vi "Subtract (Elementwise) - R,RM.vi"(1 "Real Matrix A":T1, 2 "Real Scalar c":dbl) -> (0 "c - A":T1)   [LabVIEW 2018, in "NI_Matrix.lvlib"]
doc: "Computes the difference of the inputs."
uses:
  NI_Matrix.lvlib
  RealMatrix.ctl
  Matrix To Array - RM.vi
  Array To Matrix - RA2.vi
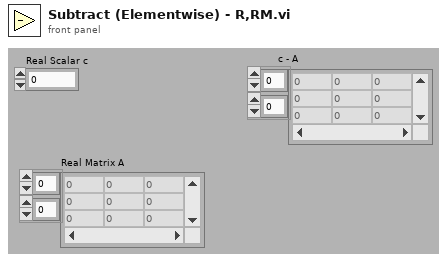
[diagram p1: front panel]
types:
  T1 = typedef "NI_Matrix.lvlib/RealMatrix.ctl" = dbl[][]
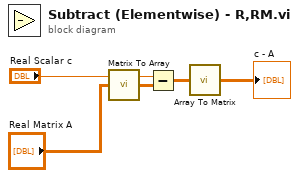
[diagram p0: block diagram]
diagram:
  n1 = call-poly "Matrix To Array.vi"("Real Matrix"="Real Matrix A") -> ("Real 2D Array"=w4:dbl[][])
  n2 = Subtract(x="Real Scalar c", y=w4) -> (x-y=w2:dbl[][])
  n3 = call-poly "Array To Matrix.vi"("Real 2D Array"=w2) -> ("Real Matrix"=→"c - A":T1)
